vi "temperature data.vi"(8 "Error In":errorcluster, 9 "append element":dbl[](array[numeric]), 10 "Input Data":dbl[][](array[numeric]), 11 "mode (R)":T1=enum."read") -> (0 "Error out":errorcluster, 2 "Output Data":dbl[][](array[numeric]))   [LabVIEW 2014]
doc: "Functional Global Variable for the algorithm settings. The used method as well as the max. Iteration steps and the tolerance can be given. In addition, the algorithm can be told to use boundaries (if possible)."
uses:
  controls/scan data action.ctl
panel:
  # "Input"
  # "Output"
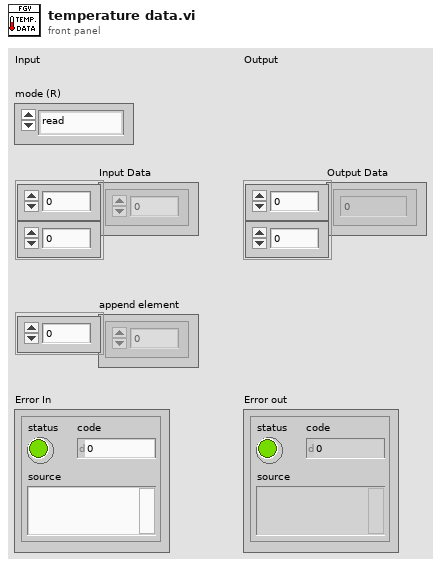
[diagram p1: front panel]
types:
  T1 = typedef "scan data action.ctl" = enum16{"initialize", "append", "read", "write"}
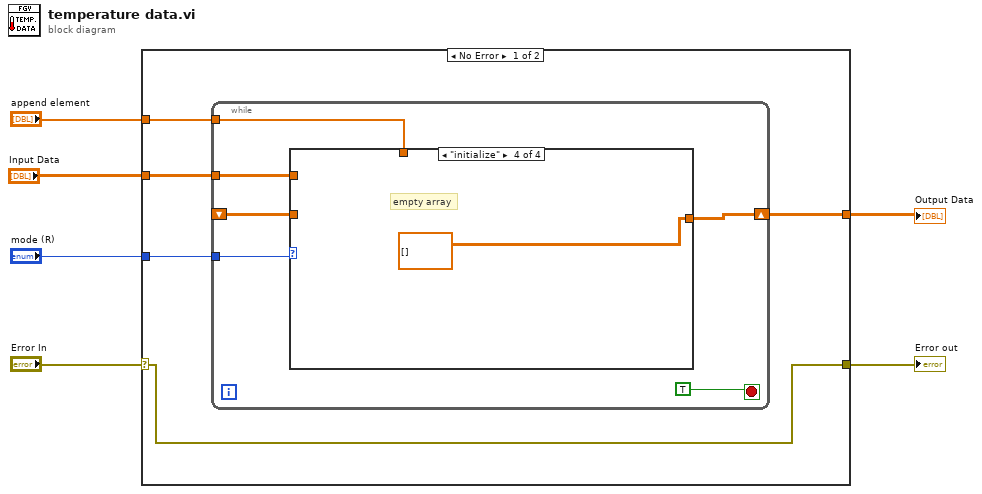
[diagram p0: block diagram]
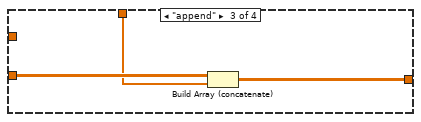
[diagram p4: hidden frame]
diagram:
  n1 = case shown="No Error" "Error In" {
    selector: "Error In" -> [w8 w25]
    tunnel: "mode (R)" -> [w11 _]
    tunnel: [w8 w25] -> w4
    tunnel: "Input Data" -> [w10 w24]
    tunnel: [w9 w24] -> w1
    tunnel: "append element" -> [w7 _]
    frame No Error {
      n2 = while {
        tunnel: w11 -> [w16]
        tunnel: w10 -> [w15]
        shift-right: [w13] -> w9
        shift-left: _ -> [w14]
        tunnel: w7 -> [w12]
        stop <- TRUE stop-if-true
        n3 = case shown="\"initialize\"" w16 {
          tunnel: w15 -> [_ w19 _ _]
          tunnel: w14 -> [w18 _ w22 _]
          tunnel: [w18 w19 w21 dbl[][] [] ("scan data Input 2")] -> w13
          tunnel: w12 -> [_ _ w20 _]
          frame "read", Default {
          }
          frame "write" {
          }
          frame "append" {
            n4 = Build Array (concatenate)(w22, w20) -> (w21:dbl[][])
          }
          frame "initialize" {
            # "empty array"
          }
        }
      }
    }
    frame Error {
    }
  }
  "Error out" <- w4
  "Output Data" <- w1
